vi "niRFUtil RFHS Channelizer Resampler.vi"(0 "Complex Waveform In":T1={"x0"=0.0, "dx"=1.0, "y"=[]} {"y" format="%.2f"; "dx" format="%^.2e"; "x0" format="%^.2e"}, 2 "CPU Context":string="M1 1", 3 "Remove Waveform Pad":bool, 5 "Target Sample Rate (Hz)":dbl=1.0 format="%#_6p", 7 "Frequence Shift (Hz)":dbl format="%#_6p", 11 "error in (no error)":errorcluster, 12 "Allowable Sampling Rate Error (ppm)":dbl=1.0 format="%_2g") -> (4 "Complex Waveform Out":T1 {"y" format="%.2f"; "dx" format="%^.2e"; "x0" format="%^.2e"}, 15 "error out":errorcluster)   [LabVIEW 2015, in "niRFUtil.lvlib"]
doc: "Wrapper for quickly using the niRFHS Channelizer as resampler."
uses:
  niRFUtil.lvlib
  Includes/niRFUtil INC Complex Waveform.ctl
  Includes/niRFUtil INC Complex Array.ctl
  Includes/niRFUtil RFHS Channelizer ChannelFlags.ctl
  Includes/niRFUtil RFHS Channelizer FilterTypeHint.ctl
  Includes/niRFUtil RFHS Channelizer ChannelSpecificationBase.ctl
  Includes/niRFUtil RFHS Channelizer ChannelSpecification.ctl
  Includes/niRFUtil RFHS Channelizer ChannelizerBufferingMode.ctl
  Utilities/niRFUtil RFHS Util Data Subset.ctl
  Includes/niRFUtil RFHS Channelizer FilterPurpose.ctl
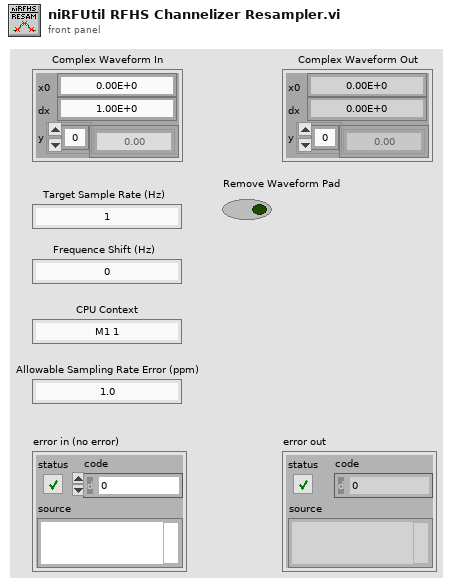
[diagram p1: front panel]
types:
  T1 = typedef "niRFUtil.lvlib/niRFUtil INC Complex Waveform.ctl" = cluster{"x0":dbl, "dx":dbl, "y":T2}
  T2 = typedef "niRFUtil.lvlib/niRFUtil INC Complex Array.ctl" = csg[]
  T3 = typedef "niRFUtil.lvlib/niRFUtil RFHS Channelizer ChannelFlags.ctl" = u32
  T4 = typedef "niRFUtil.lvlib/niRFUtil RFHS Channelizer FilterPurpose.ctl" = enum16{"Channelizer", "Fine Tune Resampler"}
  T5 = typedef "niRFUtil.lvlib/niRFUtil RFHS Util Data Subset.ctl" = cluster{"Offset":i32, "Length":i32}
  T6 = typedef "niRFUtil.lvlib/niRFUtil RFHS Channelizer ChannelizerBufferingMode.ctl" = enum32{"Unbuffered", "Finite", "Continuous"}
  T7 = typedef "niRFUtil.lvlib/niRFUtil RFHS Channelizer ChannelSpecification.ctl" = cluster{"freq in Hz":bool, "Filter Type Hint":T8, "Hint Value":dbl, "Channels":T9[]}
  T8 = typedef "niRFUtil.lvlib/niRFUtil RFHS Channelizer FilterTypeHint.ctl" = enum16{"Auto", "FFT (LTE)", "FFT (WiFi)", "FFT (custom)"}
  T9 = typedef "niRFUtil.lvlib/niRFUtil RFHS Channelizer ChannelSpecificationBase.ctl" = cluster{"fc":dbl, "fs":dbl, "passBW":dbl, "stopBW":dbl, "Rejection (dB)":dbl, "Flags":T3, "Reserved":i32}
  T10 = typedef "niRFUtil.lvlib/niRFUtil RFHS Filter Pre Post Trigger Info.ctl" = cluster{"Pre-trigger Len (input)":i64, "Min Post-trigger Len (input)":i64}
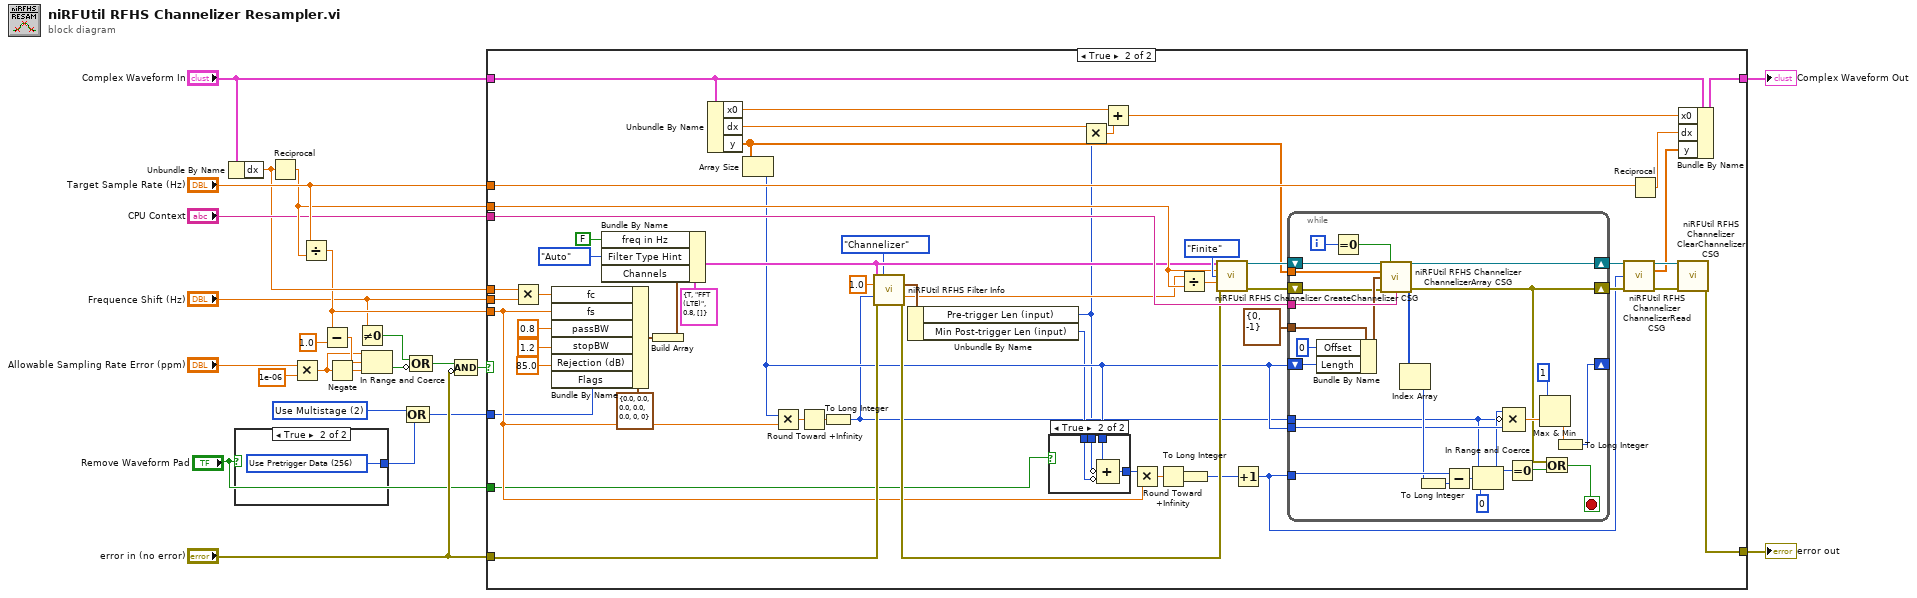
[diagram p0: block diagram]
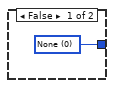
[diagram p2: hidden frame]
diagram:
  w3 = T3 2 items=["None"=0, "Force Fractional"=1, "Use Multistage"=2, "Use Pretrigger Data "=256, "Frequency Shift Only"=4] ("Flags")
  n1 = Unbundle By Name("Complex Waveform In") -> ("dx"=w18:dbl)
  n2 = case shown="True" "Remove Waveform Pad" {
    tunnel: [w25 w26] -> w4
    frame False {
      w25 = T3 0 items=["None"=0, "Force Fractional"=1, "Use Multistage"=2, "Use Pretrigger Data "=256, "Frequency Shift Only"=4] ("Flags")
    }
    frame True {
      w26 = T3 256 items=["None"=0, "Force Fractional"=1, "Use Multistage"=2, "Use Pretrigger Data "=256, "Frequency Shift Only"=4] ("Flags")
    }
  }
  n3 = Reciprocal(x=w18) -> (1/x=w21:dbl)
  n4 = Multiply(x="Allowable Sampling Rate Error (ppm)", y=1e-06 ("upper limit")) -> (x*y=w9:dbl)
  n5 = Divide(x="Target Sample Rate (Hz)", y=w21) -> (x/y=w17:dbl)
  n6 = Subtract(x=w17, y=1.0) -> (x-y=w15:dbl)
  n7 = Negate(x=w9) -> (-x=w14:dbl)
  n8 = Not Equal To 0?(x="Frequence Shift (Hz)") -> (x != 0?=w11:bool)
  n9 = In Range and Coerce(upper limit=w9, x=w15, lower limit=w14) -> (In Range?=w13:bool)  [unwired: 1 out]
  n10 = Compound Arithmetic op=OR(w3, w4) -> (w2:T3)
  n11 = Compound Arithmetic op=OR(w11, invert w13) -> (w6:bool)
  n12 = Compound Arithmetic op=AND(w6, invert "error in (no error)") -> (w5:bool)
  n13 = case shown="True" w5 {
    tunnel: "error in (no error)" -> [w28 w50]
    tunnel: [w27 w83] -> w24
    tunnel: "Complex Waveform In" -> [w27 w70]
    tunnel: "Target Sample Rate (Hz)" -> [_ w81]
    tunnel: w21 -> [_ w63]
    tunnel: "CPU Context" -> [_ w67]
    tunnel: w17 -> [_ w32]
    tunnel: [w28 w55] -> w19
    tunnel: w18 -> [_ w73]
    tunnel: "Frequence Shift (Hz)" -> [_ w72]
    tunnel: w2 -> [_ w30]
    tunnel: "Remove Waveform Pad" -> [_ w29]
    frame False {
    }
    frame True {
      n14 = Multiply(x=w73, y=w72) -> (x*y=w71:dbl)
      n15 = Bundle By Name(cluster=T9 {"fc"=0.0, "fs"=0.0, "passBW"=0.0, "stopBW"=0.0, "Rejection (dB)"=0.0, "Flags"=0, "Reserved"=0} ("Channel Spec Base"), "fc"=w71, "fs"=w32, "passBW"=0.8, "stopBW"=1.2, "Rejection (dB)"=85.0, "Flags"=w30) -> (w74:T9)
      n16 = Build Array(w74) -> (w69:T9[])
      n17 = Bundle By Name(cluster=T7 {"freq in Hz"=TRUE, "Filter Type Hint"=enum."FFT (LTE)", "Hint Value"=0.8, "Channels"=[]} ("Channel Spec"), "freq in Hz"=FALSE, "Filter Type Hint"=niRFUtil_RFHS_Channelizer_FilterTypeHint."Auto", "Channels"=w69) -> (w51:T7)
      n18 = Unbundle By Name(w70) -> ("x0"=w36:dbl, "dx"=w33:dbl, "y"=w47:T2)
      n19 = Array Size(array=w47) -> (size(s)=w46:i32)
      n20 = Multiply(x=w46, y=w32) -> (x*y=w64:dbl)
      n21 = Round Toward +Infinity(x=w64) -> (ceil(x): smallest int >= x=w57:dbl)
      n22 = To Long Integer(number=w57) -> (32bit integer=w43:i32)
      n23 = call "niRFUtil RFHS Filter Info.vi"("Channelizer Spec"=w51, "Filter Purpose"=niRFUtil_RFHS_Channelizer_FilterPurpose."Channelizer", "fs [Hz]"=1.0, "#output samples"=w43, "error in (no error)"=w50) -> ("Pre/Post Trigger Filter Info"=w45:T10, "#input samples (#output samples)"=w41:dbl, "error out"=w52:errorcluster)  [unwired: 6 in, 2 out]
      n24 = Unbundle By Name(w45) -> ("Pre-trigger Len (input)"=w39:i64, "Min Post-trigger Len (input)"=w44:i64)
      n25 = case shown="True" w29 {
        tunnel: [w84 w88] -> w48
        tunnel: w46 -> [w84 w87]
        tunnel: w44 -> [_ w86]
        tunnel: w39 -> [_ w85]
        frame False {
        }
        frame True {
          n26 = Compound Arithmetic op=ADD(w87, invert w85, invert w86) -> (w88:i64)
        }
      }
      n27 = Multiply(x=w33, y=w39) -> (x*y=w34:dbl)
      n28 = Add(x=w36, y=w34) -> (x+y=w38:dbl)
      n29 = Multiply(x=w48, y=w32) -> (x*y=w49:dbl)
      n30 = Round Toward +Infinity(x=w49) -> (ceil(x): smallest int >= x=w37:dbl)
      n31 = Divide(x=w41, y=w63) -> (x/y=w62:dbl)
      n32 = To Long Integer(number=w37) -> (32bit integer=w31:i32)
      n33 = call "niRFUtil RFHS Channelizer CreateChannelizer CSG.vi"("Channelizer Spec"=w51, "fs [Hz]"=w63, "Mode"=niRFUtil_RFHS_Channelizer_ChannelizerBufferingMode."Finite", "Buffer Size (s)"=w62, "error in (no error)"=w52) -> ("Channelizer Ref"=w66:refnum<data-value>, "error out"=w54:errorcluster)  [unwired: 9 in]
      n34 = Increment(x=w31) -> (x+1=w42:i32)
      n35 = while {
        tunnel: w47 -> [w115]
        tunnel: w67 -> [w113]
        shift-right: [w114] -> w59
        shift-left: w66 -> [w110]
        tunnel: T5 {"Offset"=0, "Length"=-1} ("Data Subset") -> [w107]
        shift-right: [w90] -> w58
        shift-left: w54 -> [w106]
        tunnel: w42 -> [w103]
        shift-right: [w99] -> _
        shift-left: w46 -> [w104]
        tunnel: w43 -> [w96]
        tunnel: w46 -> [w100]
        i -> [w109]
        stop <- w89 stop-if-true
        n36 = Bundle By Name(cluster=w107, "Offset"=0, "Length"=w104) -> (w111:T5)
        n37 = Equal To 0?(x=w109) -> (x = 0?=w108:bool)
        n38 = call "niRFUtil RFHS Channelizer ChannelizerArray CSG.vi"("Channelizer Ref"=w110, "Reset"=w108, "Data"=w115, "Data Subset"=w111, "error in (no error)"=w106, "CPU Context"=w113) -> ("Channelizer Ref (out)"=w114:refnum<data-value>, "Channel Data Len"=w105:u32[], "error out"=w90:errorcluster)  [unwired: 6 in, 1 out]
        n39 = Index Array(array=w105) -> (element=w102:u32)  [unwired: 1 in]
        n40 = To Long Integer(number=w102) -> (32bit integer=w92:i32)
        n41 = Subtract(x=w103, y=w92) -> (x-y=w97:i32)
        n42 = In Range and Coerce(upper limit=w96, x=w97, lower limit=0 ("y")) -> (coerced(x)=w98:i32)  [unwired: 1 out]
        n43 = Compound Arithmetic op=MULTIPLY(w98, invert w96, w100) -> (w93:dbl)
        n44 = Equal To 0?(x=w98) -> (x = 0?=w91:bool)
        n45 = Max & Min(x=1, y=w93) -> (max(x,y)=w94:dbl)  [unwired: 1 out]
        n46 = Or(x=w90, y=w91) -> (x .or. y?=w89:bool)
        n47 = To Long Integer(number=w94) -> (32bit integer=w99:i32)
      }
      n48 = call "niRFUtil RFHS Channelizer ChannelizerRead CSG.vi"("Channelizer Ref"=w59, "Length"=w42, "error in (no error)"=w58) -> ("Channelizer Ref (out)"=w61:refnum<data-value>, "Channel Data"=w56:csg[], "error out"=w60:errorcluster)  [unwired: 10 in]
      n49 = Reciprocal(x=w81) -> (1/x=w35:dbl)
      n50 = call "niRFUtil RFHS Channelizer ClearChannelizer CSG.vi"("Channelizer Ref"=w61, "error in (no error)"=w60) -> ("error out"=w55:errorcluster)  [unwired: 11 in, 2 out]
      n51 = Bundle By Name(cluster=w70, "x0"=w38, "dx"=w35, "y"=w56) -> (w83:T1)
    }
  }
  "error out" <- w19
  "Complex Waveform Out" <- w24
